vi "Dev List UI.vi"(8 "error in (no error)":errorcluster, 10 "stop event":refnum<user-event>, 11 "Operator UI in":refnum<class "Controller UI.lvclass">) -> (0 "error out":errorcluster)   [LabVIEW 2016, in "Controller UI.lvlib" / "Controller UI.lvclass"]
uses:
  <userlib>/Common Components/Controller UI/Controller UI.lvclass
  System.Windows.Forms
  C:/Program Files (x86)/National Instruments/LabVIEW 2016/vi.lib/ActorFramework/Actor/Actor.lvclass
  <userlib>/LabVIEWdotNetDataGrid/source/GridColumn/ColumnDefinition.ctl
  <userlib>/LabVIEWdotNetDataGrid/source/GridColumn/ColumnType.ctl
  <userlib>/Common Components/Controller UI/Controller UI.lvclass/Controller UI.ctl
  <vilib>/ActorFramework/Actor/Actor.lvclass/Actor.ctl
  <vilib>/ActorFramework/Message Enqueuer/Message Enqueuer.lvclass/Message Enqueuer.ctl
  <userlib>/Common Components/Hardware/DevInfo/DTColumn Index.ctl
  <userlib>/Common Components/Controller UI/Dev Variant Data.ctl
  <userlib>/Common Components/Hardware/DevInfo/DevInfo.lvclass
  <userlib>/Common Components/Controller UI/Update DT event data - checked out.ctl
  <userlib>/Common Components/Controller UI/Update DT event data - COMM status.ctl
  <userlib>/Common Components/Controller UI/DT Data File.ctl
  <userlib>/Common Components/Controller UI Messages/Write Selected DTRows Msg/Write Selected DTRows Msg.lvclass/Write Selected DTRows Msg.ctl
  <userlib>/Common Components/Controller Messages/Check Fcn and Dev Selection requested by UI Msg/Check Fcn and Dev Selection requested by UI Msg.lvclass/Check Fcn and Dev Selection requested by UI Msg.ctl
  <vilib>/Utility/error.llb/DialogType.ctl
  <userlib>/Common Components/Controller UI/Accessors/Read Update DT event.vi
  <userlib>/Common Components/Controller UI/Accessors/Read Function.vi
  <userlib>/Common Components/Controller UI/Accessors/Read Master_Slave.vi
  <vilib>/ActorFramework/Message Enqueuer/Init from Existing Queue.vi
  <vilib>/ActorFramework/Message Enqueuer/Enqueue.vi
  <userlib>/Common Components/Controller Messages/Check Fcn and Dev Selection requested by UI Msg/Check Fcn and Dev Selection requested by UI Msg.lvclass
  C:/Program Files (x86)/National Instruments/LabVIEW 2016/vi.lib/ActorFramework/Message/Message.lvclass
  <userlib>/Common Components/Controller UI Messages/Write Selected DTRows Msg/Write Selected DTRows Msg.lvclass
  <userlib>/Common Components/Controller Messages/Update Available COMM List Msg/Update Available COMM List Msg.lvclass
  <userlib>/LabVIEWdotNetDataGrid/source/DataGridView/Set DataCell (String).vi
  <vilib>/Utility/xml.llb/Read From XML File(string).vi
  <userlib>/LabVIEWdotNetDataGrid/source/DataGridView/Get DataArray (String).vi
  <vilib>/Utility/xml.llb/Write to XML File(string).vi
  <userlib>/LabVIEWdotNetDataGrid/source/DataGridView/Set ComboCell DataSource (String).vi
  <vilib>/ActorFramework/Message Priority Queue/Priority Enqueue.vi
  <vilib>/ActorFramework/Message Enqueuer/Message Enqueuer.lvclass
  <userlib>/LabVIEWdotNetDataGrid/source/DataGrid.lvlib
  <userlib>/LabVIEWdotNetDataGrid/source/Events/CellValueChanged/CellValueChanged.lvclass
  <userlib>/LabVIEWdotNetDataGrid/source/Events/CellClick/CellClick.lvclass
  <userlib>/LabVIEWdotNetDataGrid/source/Events/KeyDown/KeyDown.lvclass
  <userlib>/LabVIEWdotNetDataGrid/source/DataGridView/DataGridView.lvclass
  <userlib>/LabVIEWdotNetDataGrid/source/GridColumn/GridColumn.lvclass
  <vilib>/ActorFramework/Actor/Actor.lvclass
  <userlib>/LabVIEWdotNetDataGrid/source/DataTable/DataTable.lvclass
  <userlib>/Common Components/Common/Common.lvlib
  <userlib>/Common Components/Controller/Messages/Log Status/Log Status.lvclass
panel:
  in  "Refresh Button":bool
  in  "Down Button":bool
  in  "Up Button":bool
  in  "Remove Button":bool
  in  "Insert Button":bool
  in  "HW/DEV list":refnum<k24>(container)
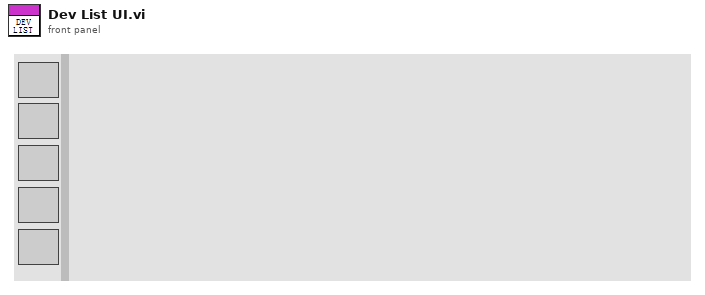
[diagram p1: front panel]
types:
  T1 = typedef "DataGrid.lvlib/GridColumn.lvclass/ColumnDefinition.ctl" = cluster{"name":string, "caption":string, "datatype":T2, "Params":string, "AutoSizeMode":i32, "FillWeight":sgl, "MinWidth":u32, "tooltip":string, "ReadOnly?":bool, "Visible?":bool}
  T2 = typedef "DataGrid.lvlib/GridColumn.lvclass/ColumnType.ctl" = enum16{"string", "image", "check", "numeric", "timestamp", "button", "combo", "link"}
  T3 = cluster{"registeredEvents":refnum<event-registration>, "Event Registration Refnum":refnum<event-registration>}
  T4 = typedef "Hardware.lvlib/DevInfo.lvclass/DTColumn Index.ctl" = enum16{"GUID", "Check", "Checked-out", "Status", "Device", "Label", "COMM", "Sub-COMM", "COMM Settings"}
  T5 = typedef "Controller UI.lvlib/Controller UI.lvclass/Update DT event data - checked out.ctl" = cluster{"GUID":string, "checked-out?":bool}
  T6 = typedef "Controller UI.lvlib/Controller UI.lvclass/Dev Variant Data.ctl" = cluster{"Row Index":i32, "DevInfo Obj":refnum<class "DevInfo.lvclass">}
  T7 = typedef "Controller UI.lvlib/Controller UI.lvclass/Update DT event data - COMM status.ctl" = cluster{"GUID":string, "COMM status":bool}
  T8 = typedef "Controller UI.lvlib/Controller UI.lvclass/DT Data File.ctl" = cluster{"ColumnSetup":T1[], "DataArray":string[][]}
  T9 = typedef "Controller UI.lvlib/Controller UI.lvclass/Update DT Cmd.ctl" = enum16{"Update HWtype\\HWplugin array", "Update Checked-out", "Update COMM Status", "Load DevInfo from File", "Save DevInfo to File", "Update COMM Address List"}
  T10 = typedef "DialogType.ctl" = u16
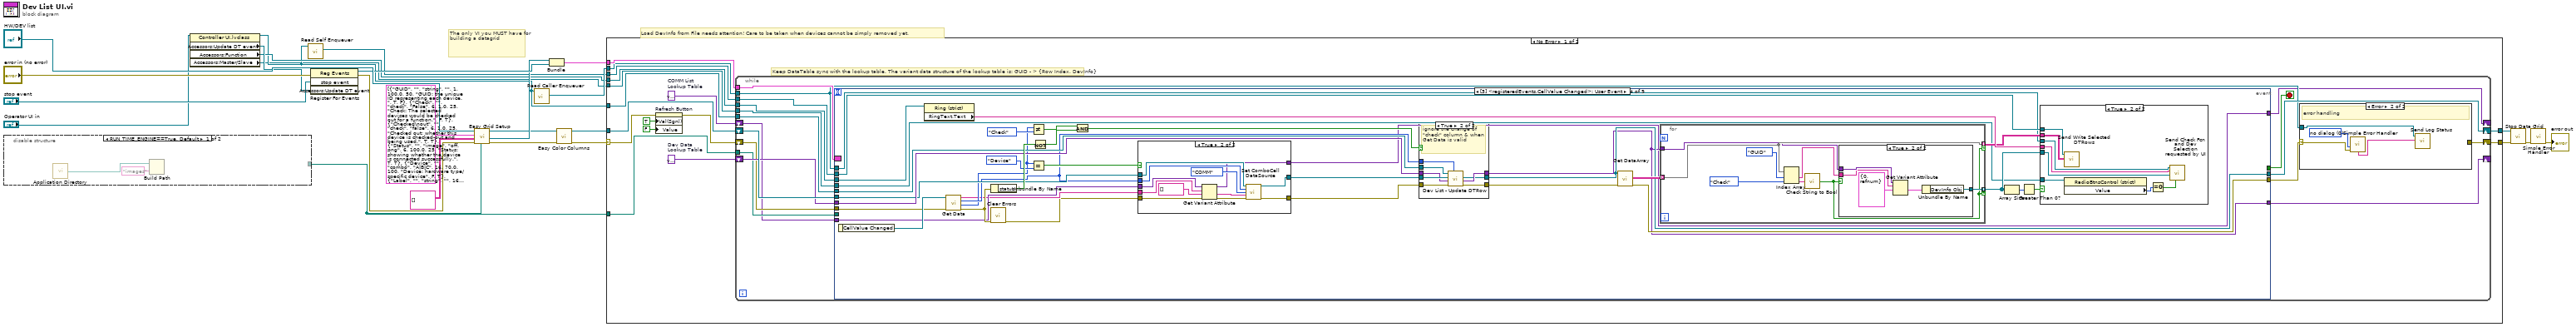
[diagram p0: block diagram]
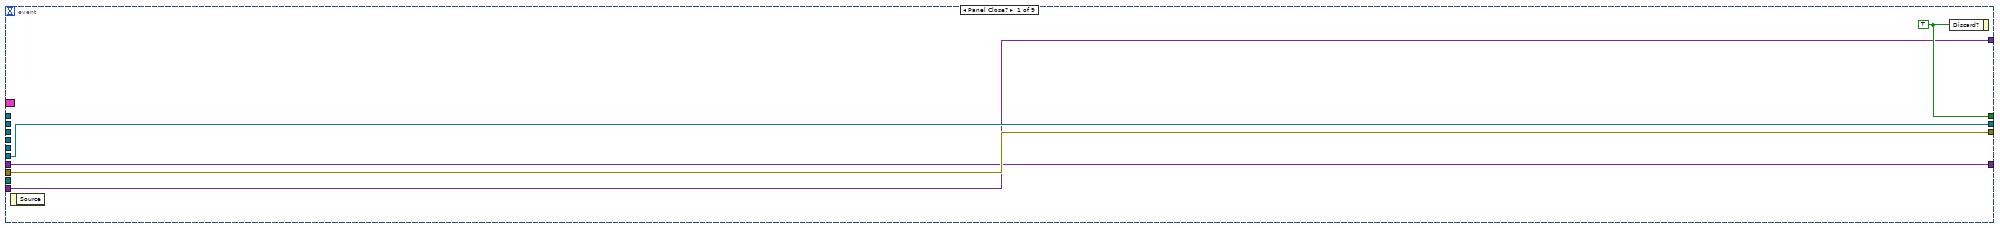
[diagram p3: hidden frame]
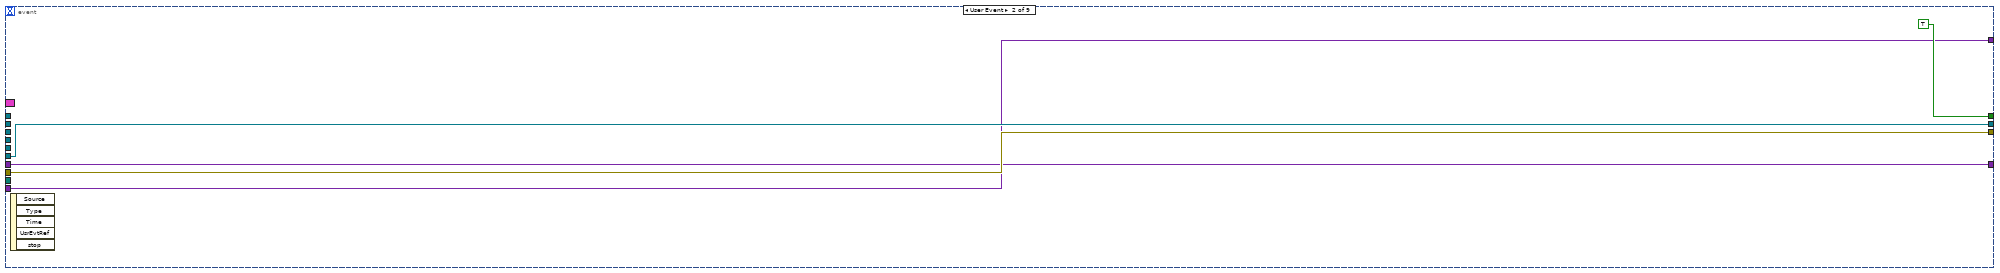
[diagram p4: hidden frame]
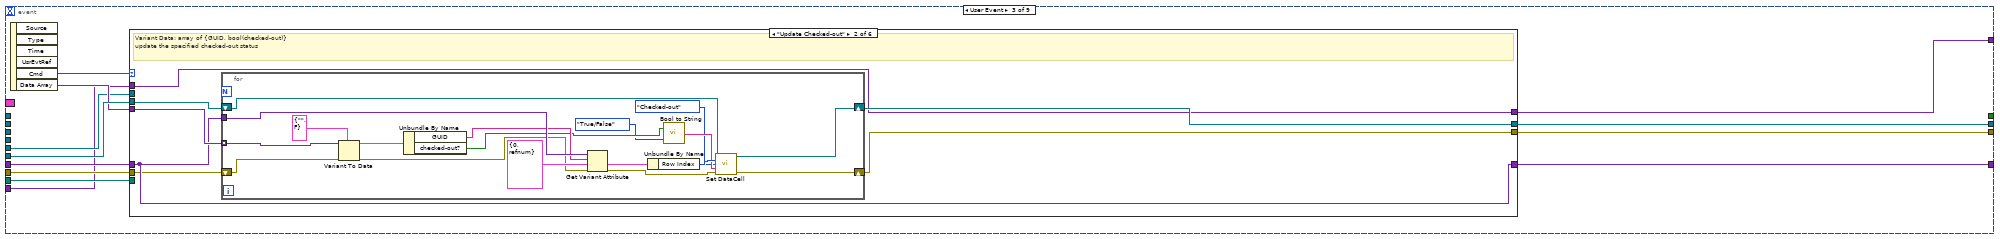
[diagram p5: hidden frame]
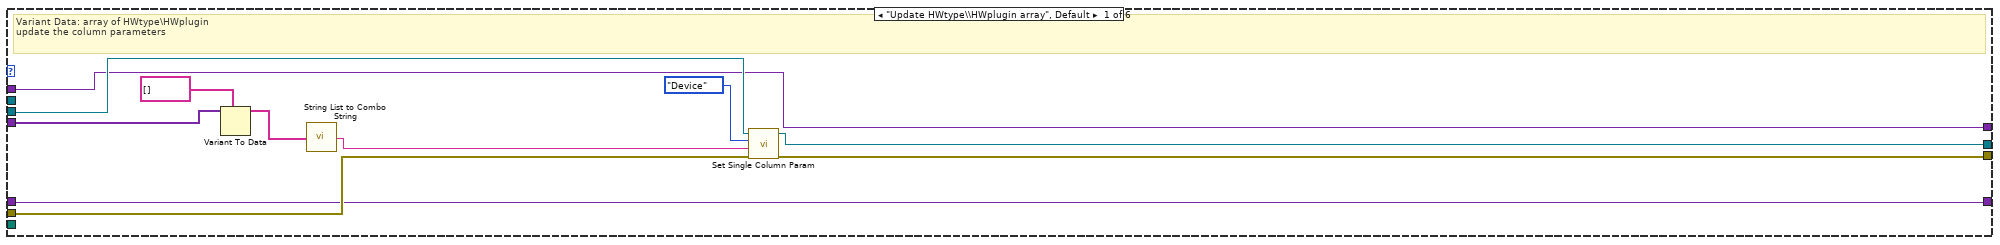
[diagram p6: hidden frame]
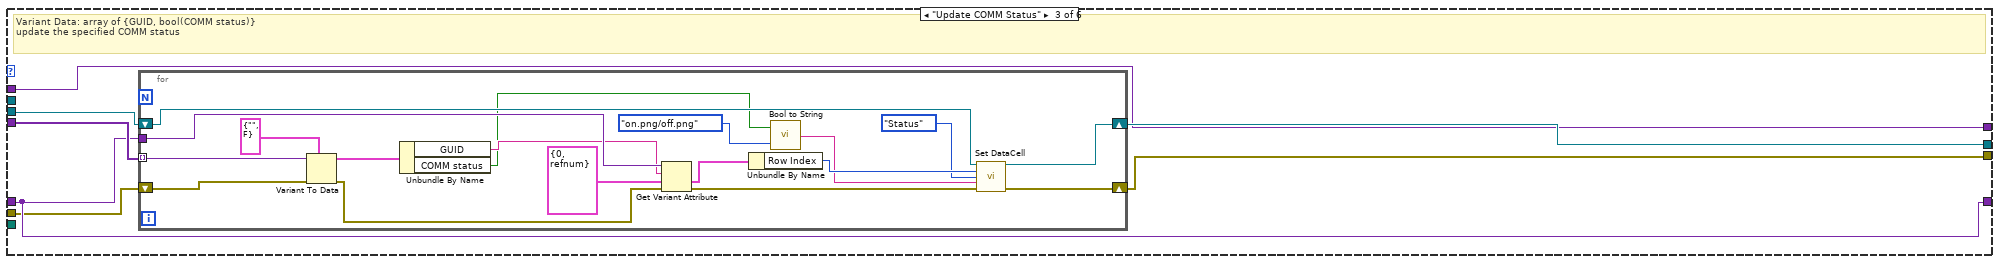
[diagram p7: hidden frame]
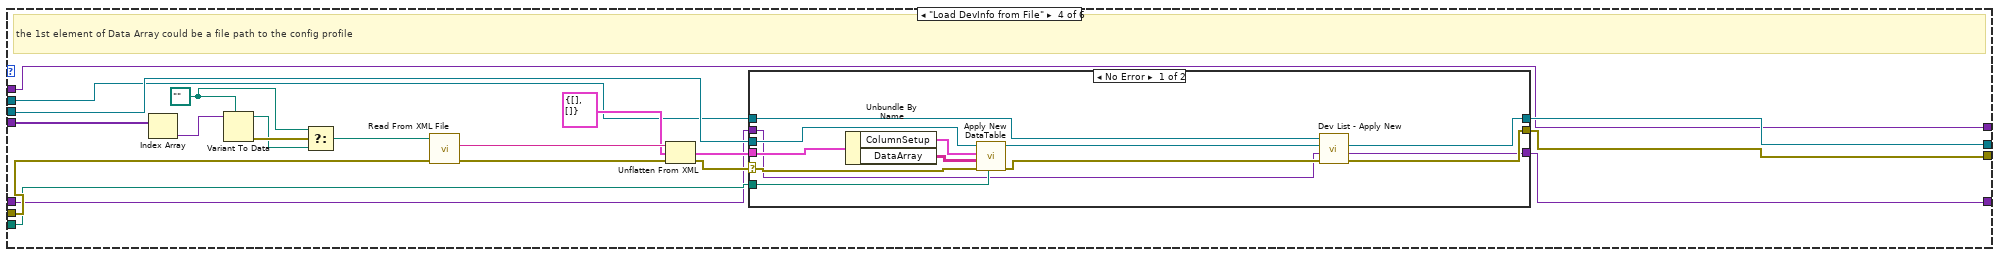
[diagram p8: hidden frame]
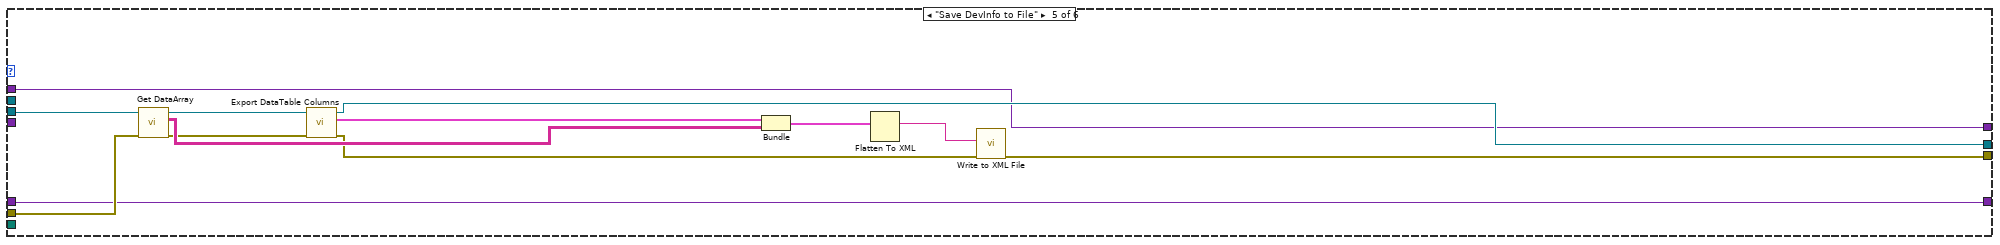
[diagram p10: hidden frame]
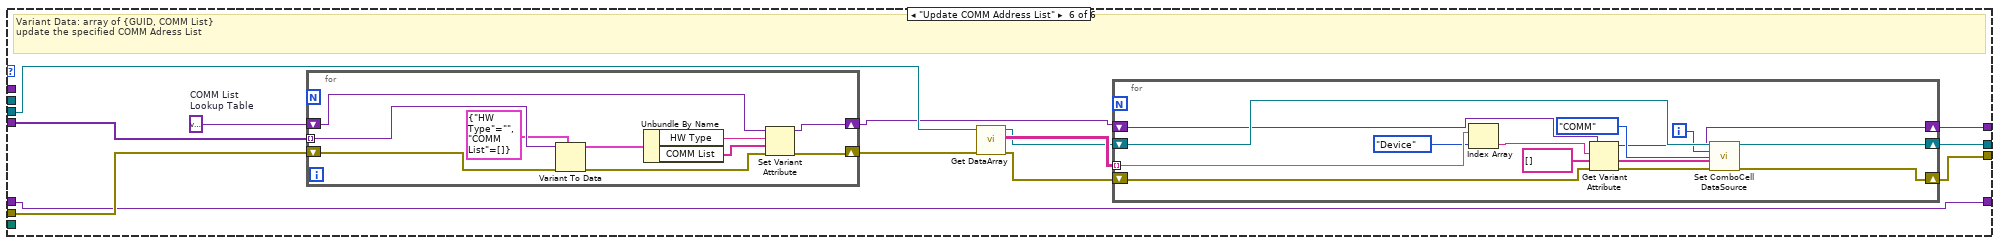
[diagram p11: hidden frame]
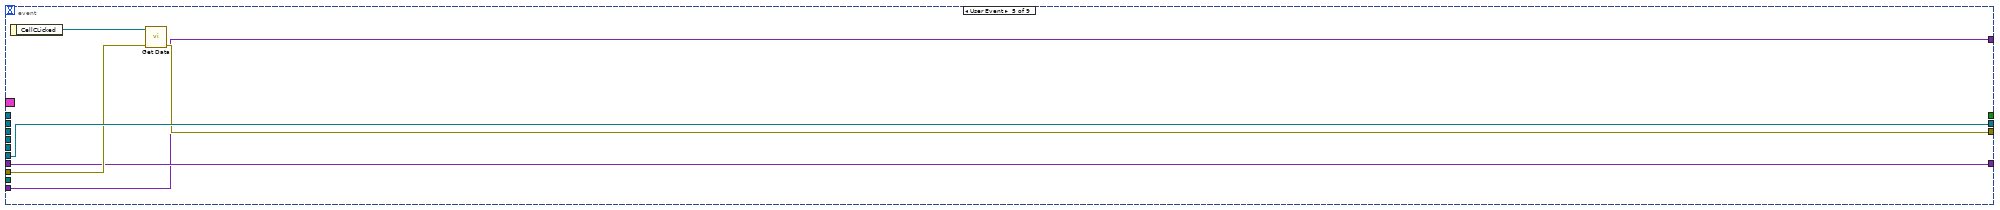
[diagram p16: hidden frame]
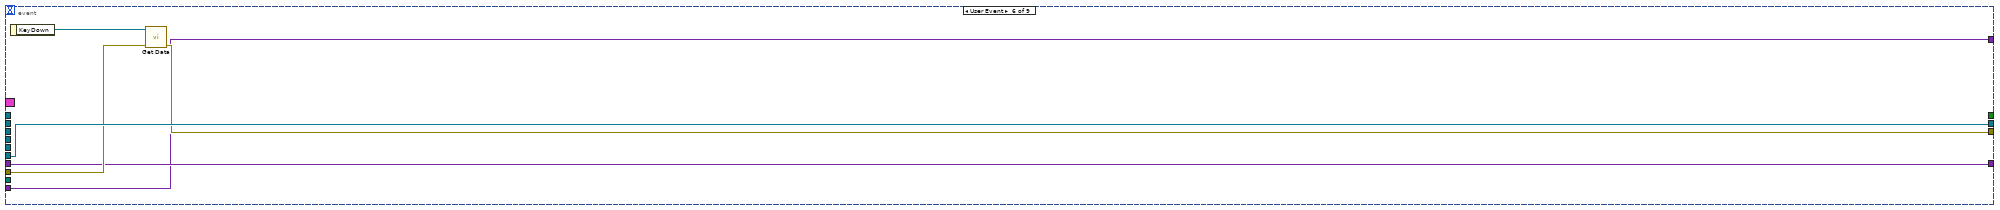
[diagram p17: hidden frame]
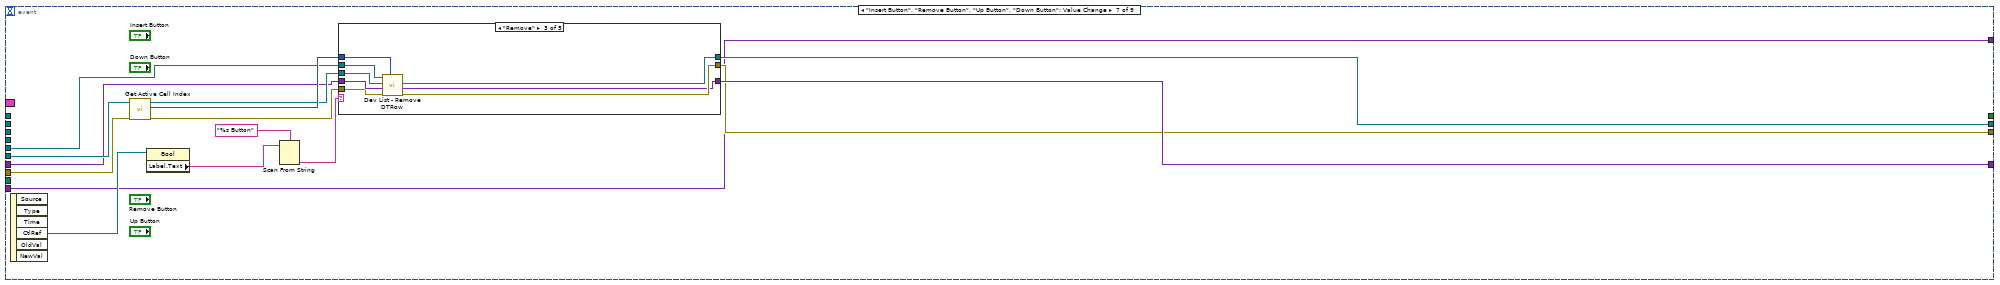
[diagram p18: hidden frame]
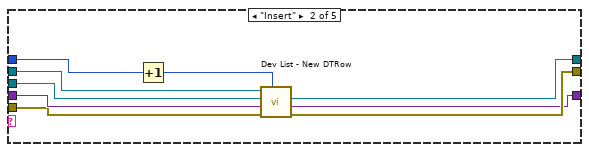
[diagram p20: hidden frame]
diagram:
  # "Load DevInfo from File needs attention! Care to be taken when devices cannot be simply removed yet."
  # "The only VI you MUST have for building a datagrid"
  n1 = disable-structure shown="RUN_TIME_ENGINE==True, Default" {
    disable-tunnel: [_ path "C:/Program Files (x86)/National Instruments/LabVIEW 2016/user.lib/LabVIEWdotNetDataGrid/images"] -> w2
    frame condition #0 {
      n2 = call <vilib>:"Application Directory.vi"() -> ("Application Directory"=w27:path)
      n3 = Build Path(base path=w27, name or relative path="images") -> ()  [unwired: 1 out]
    }
    frame condition #1 (active) {
    }
  }
  n4 = property class="Controller UI.lvclass"(reference="Operator UI in") -> (reference out=w6:refnum<class "Controller UI.lvclass">, "Accessors:Update DT event"=w9:refnum<user-event>, "Accessors:Function"=w7:refnum<vi>, "Accessors:Master/Slave"=w1:refnum<vi>)  [unwired: 1 in, 1 out]
  n5 = call <vilib>:"Read Self Enqueuer.vi"("Actor"=w6) -> ("Self Enqueuer"=w8:refnum<class "Message Enqueuer.lvclass">)  [unwired: 10 in]
  n6 = register-events(error in="error in (no error)", "stop event", w9) -> (reference out=w19:refnum<event-registration>, error out=w15:errorcluster)  [unwired: 1 in]
  n7 = call <userlib>:"Easy Grid Setup.vi"("Images Path"=w2, "error in"=w15, "DataSource Data"=string[][] [], "ColumnSetup"=T1[] [{"name"="GUID", "caption"="", "datatype"=enum."string", "Params"="", "AutoSizeMode"=1, "FillWeight"=100.0, "MinWidth"=50, "tooltip"="GUID: the unique ID representing each device.", "ReadOnly?"=TRUE, "Visible?"=FALSE}, {"name"="Check", "caption"="", "datatype"=enum."check", "Params"="False", "AutoSizeMode"=6, "FillWeight"=1.0, "MinWidth"=25, "tooltip"="Check: The selected devices would be checked out for a function.", "ReadOnly?"=FALSE, "Visible?"=TRUE}, {"name"="Checked\nout", "caption"="", "datatype"=enum."check", "Params"="false", "AutoSizeMode"=6, "FillWeight"=1.0, "MinWidth"=25, "tooltip"="Checked out: whether this device is checked-out and being used.", "ReadOnly?"=TRUE, "Visible?"=TRUE}, {"name"="Status", "caption"="", "datatype"=enum."image", "Params"="off.png", "AutoSizeMode"=6, "FillWeight"=100.0, "MinWidth"=25, "tooltip"="Status: showing whether the device is connected successfully.", "ReadOnly?"=TRUE, "Visible?"=TRUE}, {"name"="Device", "caption"="", "datatype"=enum."combo", "Params"="A|B|C", "AutoSizeMode"=16, "FillWeight"=70.0, "MinWidth"=100, "tooltip"="Device: hardware type/specific device", "ReadOnly?"=FALSE, "Visible?"=TRUE}, {"name"="Label", "caption"="", "datatype"=enum."string", "Params"="", "AutoSizeMode"=16, "FillWeight"=30.0, "MinWidth"=50, "tooltip"="Label: used as the alias in a running function, so multiple devices of the same abstract hardware type should have different labels in the same running function.", "ReadOnly?"=FALSE, "Visible?"=TRUE}, {"name"="COMM", "caption"="", "datatype"=enum."combo", "Params"="", "AutoSizeMode"=6, "FillWeight"=1.0, "MinWidth"=30, "tooltip"="COMM: the main communication port, e.g. COM, CAN ID, etc.", "ReadOnly?"=FALSE, "Visible?"=TRUE}, {"name"="Sub-\nCOMM", "caption"="", "datatype"=enum."numeric", "Params"="", "AutoSizeMode"=4, "FillWeight"=1.0, "MinWidth"=60, "tooltip"="Sub-COMM: address to the device if multiple connected to the main COMM.", "ReadOnly?"=FALSE, "Visible?"=TRUE}, {"name"="COMM\nSettings", "caption"="", "datatype"=enum."button", "Params"="", "AutoSizeMode"=6, "FillWeight"=1.0, "MinWidth"=20, "tooltip"="COMM Settings: clickable button if such settings available.", "ReadOnly?"=FALSE, "Visible?"=TRUE}], "DataGridView"="HW/DEV list") -> ("error out"=w25:errorcluster, "registeredEvents"=w18:refnum<event-registration>, "DataGrid out"=w5:refnum<class "DataGridView.lvclass">)  [unwired: 3 in, 1 out]
  n8 = call <vilib>:"Read Caller Enqueuer.vi"("Actor"=w6) -> ("Caller Enqueuer"=w11:refnum<class "Message Enqueuer.lvclass">)  [unwired: 10 in]
  n9 = Bundle("registeredEvents"=w18, "Event Registration Refnum"=w19) -> (w17:T3)  [unwired: 1 in]
  n10 = call <userlib>:"Easy Color Columns.vi"("error in (no error)"=w25, "DataGridView in"=w5) -> ("error out"=w4:errorcluster, "DataGridView out"=w24:refnum<class "DataGridView.lvclass">)  [unwired: 8 in]
  n11 = case shown="No Error" w4 {
    selector: w4 -> [w33 w382]
    tunnel: w24 -> [w44 w381]
    tunnel: [w43 w381] -> w23
    tunnel: w17 -> [w42 _]
    tunnel: [w41 w382] -> w3
    tunnel: w11 -> [w40 _]
    tunnel: w8 -> [w39 _]
    tunnel: w7 -> [w38 _]
    tunnel: w6 -> [w36 _]
    tunnel: w2 -> [w31 _]
    tunnel: w1 -> [w29 _]
    frame No Error {
      w30 = variant  # COMM List Lookup Table
      w37 = variant  # Dev Data Lookup Table
      # "Keep DataTable sync with the lookup table. The variant data structure of the lookup table is: GUID - > {Row Index, DevInfo}"
      n12 = property on="Refresh Button" class="Bool (strict)"(error in=w33, "Val(Sgnl)"=TRUE, "Value"=FALSE) -> (error out=w32:errorcluster)  [unwired: 1 in, 1 out]
      n13 = while {
        shift-right: [w60] -> w43
        shift-left: w44 -> [w61]
        tunnel: w42 -> [w59]
        tunnel: w40 -> [w48]
        tunnel: w39 -> [w57]
        tunnel: w38 -> [w56]
        shift-right: [w54] -> _
        shift-left: w37 -> [w55]
        tunnel: w36 -> [w53]
        shift-right: [w51] -> w41
        shift-left: w32 -> [w50]
        tunnel: w31 -> [w49]
        shift-right: [w46] -> _
        shift-left: w30 -> [w47]
        tunnel: w29 -> [w45]
        stop <- w58 stop-if-true
        n14 = event shown="[3] <registeredEvents.CellValue Changed>: User Event" {
          selector: w59 -> [_ _ _ _ _ _ _ _ _]
          dyn-events: _ -> [_ _ _ _ _ _ _ _ _]
          timeout: _ -> [_ _ _ _ _ _ _ _ _]
          tunnel: [w71 TRUE _ _ _ _ _ _ _] -> w58
          tunnel: w61 -> [w70 w76 w88 w246 w323 w329 w340 w375 w380]
          tunnel: [w70 w76 w85 w266 w323 w329 w338 w375 w380] -> w60
          tunnel: [w69 w75 w86 w263 w321 w327 w332 w373 w379] -> w52
          tunnel: w50 -> [w69 w75 w87 w269 w320 w326 w339 w373 w379]
          tunnel: w48 -> [_ _ _ w237 _ _ _ w371 _]
          tunnel: w57 -> [_ _ _ w268 _ _ _ _ _]
          tunnel: w56 -> [_ _ _ w265 _ _ _ _ _]
          tunnel: w55 -> [w68 w73 w82 w251 w319 w325 w335 w374 w378]
          tunnel: [w68 w73 w80 w249 w319 w325 w334 w374 w378] -> w54
          tunnel: w53 -> [_ _ w79 w250 _ _ w333 _ _]
          tunnel: w49 -> [_ _ w81 _ _ _ _ _ _]
          tunnel: w47 -> [w67 w72 w78 w243 w318 w324 w330 w372 w376]
          tunnel: [w67 w72 w77 w242 w318 w324 w330 w372 w376] -> w46
          tunnel: w45 -> [_ _ _ w236 _ _ _ _ _]
          event Panel Close? {
            w71 = TRUE ("Discard?")
            n15 = event-data() -> ()  [unwired: 1 in, 1 out]
            n16 = event-data("Discard?"=w71) -> ()  [unwired: 1 in, 1 out]
          }
          event User Event {
            n17 = event-data() -> ()  [unwired: 1 in, 5 out]
          }
          event User Event {
            n18 = event-data() -> ("Cmd"=w83:T9, "Data Array"=w84:variant[])  [unwired: 1 in, 4 out]
            n19 = case shown="\"Update Checked-out\"" w83 {
              tunnel: w88 -> [w99 w104 w129 w161 w198 w206]
              tunnel: w87 -> [w98 w102 w127 w166 w191 w211]
              tunnel: [w97 w101 w126 w163 w188 w199] -> w86
              tunnel: [w96 w103 w128 w162 w192 w203] -> w85
              tunnel: w84 -> [w95 w106 w131 w156 _ w210]
              tunnel: w82 -> [w90 w105 w130 w159 w187 w209]
              tunnel: w81 -> [_ _ _ w160 _ _]
              tunnel: [w90 w105 w130 w158 w187 w209] -> w80
              tunnel: w79 -> [_ _ _ w157 _ _]
              tunnel: w78 -> [w89 w100 w125 w150 w186 _]
              tunnel: [w89 w100 w125 w150 w186 w201] -> w77
              frame "Update HWtype\\HWplugin array", Default {
                # "Variant Data: array of HWtype\\HWplugin\nupdate the column parameters"
                n20 = Variant To Data(type=string[] [], Variant=w95) -> (data=w92:string[])  [unwired: 1 in, 1 out]
                n21 = call <userlib>:"String List to Combo String.vi"("find list"=w92) -> ("String"=w91:string)
                n22 = call <userlib>:"Set Single Column Param.vi"("error in (no error)"=w98, "Params"=w91, "column index"=DTColumn_Index."Device" ("DTColumn Index"), "DataGridView in"=w99) -> ("error out"=w97:errorcluster, "DataGridView out"=w96:refnum<class "DataGridView.lvclass">)  [unwired: 6 in]
              }
              frame "Update Checked-out" {
                # "Variant Data: array of {GUID, bool(checked-out)}\nupdate the specified checked-out status"
                n23 = for {
                  tunnel: w106 -> [w123] mode=indexing
                  tunnel: w105 -> [w124]
                  shift-right: [w118] -> w103
                  shift-left: w104 -> [w119]
                  shift-right: [w113] -> w101
                  shift-left: w102 -> [w111]
                  n24 = Variant To Data(error in=w111, type=T5 {"GUID"="", "checked-out?"=FALSE}, Variant=w123) -> (data=w112:T5, error out=w110:errorcluster)
                  n25 = Unbundle By Name(w112) -> ("GUID"=w122:string, "checked-out?"=w116:bool)
                  n26 = Get Variant Attribute(Variant=w124, name=w122, default value (empty Variant)=T6 {"Row Index"=0, "DevInfo Obj"=refnum} ("Dev Variant Data"), error in=w110) -> (value=w120:T6, error out=w114:errorcluster)  [unwired: 2 out]
                  n27 = Unbundle By Name(w120) -> ("Row Index"=w117:i32)
                  n28 = call <userlib>:"Bool to String.vi"("type (True/False)"=enum16{"True/False", "on.png/off.png"}."True/False", "Boolean"=w116) -> ("Bool String"=w115:string)
                  n29 = call-poly <userlib>:"Set DataCell.vi"("DataGridView in"=w119, "row index"=w117, "col index"=DTColumn_Index."Checked-out" ("DTColumn Index"), "Data"=w115, "error in"=w114) -> ("DataGridView out"=w118:refnum<class "DataGridView.lvclass">, "error out"=w113:errorcluster)  [unwired: 9 in]
                }
              }
              frame "Update COMM Status" {
                # "Variant Data: array of {GUID, bool(COMM status)}\nupdate the specified COMM status"
                n30 = for {
                  tunnel: w131 -> [w148] mode=indexing
                  tunnel: w130 -> [w149]
                  shift-right: [w143] -> w128
                  shift-left: w129 -> [w144]
                  shift-right: [w138] -> w126
                  shift-left: w127 -> [w136]
                  n31 = Variant To Data(error in=w136, type=T7 {"GUID"="", "COMM status"=FALSE} ("Cluster"), Variant=w148) -> (data=w137:T7, error out=w135:errorcluster)
                  n32 = Unbundle By Name(w137) -> ("GUID"=w147:string, "COMM status"=w141:bool)
                  n33 = Get Variant Attribute(Variant=w149, name=w147, default value (empty Variant)=T6 {"Row Index"=0, "DevInfo Obj"=refnum} ("Dev Variant Data"), error in=w135) -> (value=w145:T6, error out=w139:errorcluster)  [unwired: 2 out]
                  n34 = Unbundle By Name(w145) -> ("Row Index"=w142:i32)
                  n35 = call <userlib>:"Bool to String.vi"("type (True/False)"=enum16{"True/False", "on.png/off.png"}."on.png/off.png", "Boolean"=w141) -> ("Bool String"=w140:string)
                  n36 = call-poly <userlib>:"Set DataCell.vi"("DataGridView in"=w144, "row index"=w142, "col index"=DTColumn_Index."Status" ("DTColumn Index"), "Data"=w140, "error in"=w139) -> ("DataGridView out"=w143:refnum<class "DataGridView.lvclass">, "error out"=w138:errorcluster)  [unwired: 9 in]
                }
              }
              frame "Load DevInfo from File" {
                w152 = path "" ("XML File Path")
                # "the 1st element of Data Array could be a file path to the config profile"
                n37 = Index Array(array=w156) -> (element=w155:variant)  [unwired: 1 in]
                n38 = Variant To Data(type=w152, Variant=w155) -> (data=w153:path, error out=w154:errorcluster)  [unwired: 1 in]
                n39 = Select(t=w152, s=w154, f=w153) -> (s? t:f=w151:path)
                n40 = call-poly <vilib>:"Read From XML File.vi"("error in (no error)"=w166, "XML File Path"=w151) -> ("error out"=w165:errorcluster, "XML Elements"=w169:string)  [unwired: 7 in, 1 out]
                n41 = Unflatten From XML(xml string=w169, type=T8 {"ColumnSetup"=[], "DataArray"=[]} ("output cluster"), error in (no error)=w165) -> (value=w167:T8, error out=w164:errorcluster)
                n42 = case shown="No Error" w164 {
                  selector: w164 -> [w177 w184]
                  tunnel: w167 -> [w182 _]
                  tunnel: [w175 w184] -> w163
                  tunnel: [w173 w185] -> w162
                  tunnel: w161 -> [w179 w185]
                  tunnel: w160 -> [w178 _]
                  tunnel: w159 -> [w172 w183]
                  tunnel: [w171 w183] -> w158
                  tunnel: w157 -> [w170 _]
                  frame No Error {
                    n43 = Unbundle By Name(w182) -> ("ColumnSetup"=w181:T1[], "DataArray"=w180:string[][])
                    n44 = call <userlib>:"Apply New DataTable.vi"("Images Path"=w178, "error in (no error)"=w177, "DataArray"=w180, "ColumnSetup"=w181, "DataGridView in"=w179) -> ("error out"=w176:errorcluster, "DataGridView out"=w174:refnum<class "DataGridView.lvclass">)  [unwired: 5 in]
                    n45 = call <userlib>:"Dev List - Apply New.vi"("error in (no error)"=w176, "Dev Data Lookup Table in"=w172, "DataGridView in"=w174, "Controller UI in"=w170) -> ("error out"=w175:errorcluster, "Dev Data Lookup Table in out"=w171:variant, "DataGridView out"=w173:refnum<class "DataGridView.lvclass">)  [unwired: 5 in]
                  }
                  frame Error {
                  }
                }
              }
              frame "Save DevInfo to File" {
                n46 = call-poly <userlib>:"Get DataArray.vi"("error in (no error)"=w191, "DataGridView in"=w198) -> ("error out"=w190:errorcluster, "Array"=w195:string[][], "DataGridView out"=w197:refnum<class "DataGridView.lvclass">)  [unwired: 7 in]
                n47 = call <userlib>:"Export DataTable Columns.vi"("error in (no error)"=w190, "DataGridView in"=w197) -> ("error out"=w189:errorcluster, "ColumnSetup"=w196:T1[], "DataGridView out"=w192:refnum<class "DataGridView.lvclass">)  [unwired: 7 in]
                n48 = Bundle("ColumnSetup"=w196, "Array"=w195) -> (w194:cluster{"ColumnSetup":T1[], "Array":string[][]})  [unwired: 1 in]
                n49 = Flatten To XML(anything=w194) -> (xml string=w193:string)
                n50 = call-poly <vilib>:"Write to XML File.vi"("error in (no error)"=w189, "XML Input"=w193) -> ("error out"=w188:errorcluster)  [unwired: 7 in, 2 out]
              }
              frame "Update COMM Address List" {
                w207 = variant  # COMM List Lookup Table
                # "Variant Data: array of {GUID, COMM List}\nupdate the specified COMM Adress List"
                n51 = for {
                  tunnel: w210 -> [w234] mode=indexing
                  shift-right: [w232] -> w208
                  shift-left: w211 -> [w230]
                  shift-right: [w226] -> w202
                  shift-left: w207 -> [w235]
                  n52 = Variant To Data(error in=w230, type=cluster{"HW Type":string, "COMM List":string[]} {"HW Type"="", "COMM List"=[]} ("Cluster"), Variant=w234) -> (data=w231:cluster{"HW Type":string, "COMM List":string[]}, error out=w229:errorcluster)
                  n53 = Unbundle By Name(w231) -> ("HW Type"=w233:string, "COMM List"=w227:string[])
                  n54 = Set Variant Attribute(Variant=w235, name=w233, value=w227, error in=w229) -> (Variant out=w226:variant, error out=w232:errorcluster)  [unwired: 1 out]
                }
                n55 = call-poly <userlib>:"Get DataArray.vi"("error in (no error)"=w208, "DataGridView in"=w206) -> ("error out"=w200:errorcluster, "Array"=w205:string[][], "DataGridView out"=w204:refnum<class "DataGridView.lvclass">)  [unwired: 7 in]
                n56 = for {
                  tunnel: w205 -> [w221] mode=indexing
                  shift-right: [w224] -> w203
                  shift-left: w204 -> [w225]
                  shift-right: [w215] -> w201
                  shift-left: w202 -> [w219]
                  shift-right: [w212] -> w199
                  shift-left: w200 -> [w214]
                  i -> [w223]
                  n57 = Index Array(array=w221, index=DTColumn_Index."Device" ("DTColumn Index")) -> (element=w218:string)
                  n58 = Get Variant Attribute(Variant=w219, name=w218, default value (empty Variant)=string[] [] ("COMM List"), error in=w214) -> (duplicate Variant=w215:variant, value=w216:string[], error out=w213:errorcluster)  [unwired: 1 out]
                  n59 = call-poly <userlib>:"Set ComboCell DataSource.vi"("DataGridView in"=w225, "row index"=w223, "col index"=DTColumn_Index."COMM" ("DTColumn Index"), "Combo DataSource"=w216, "error in"=w213) -> ("DataGridView out"=w224:refnum<class "DataGridView.lvclass">, "error out"=w212:errorcluster)  [unwired: 9 in]
                }
              }
            }
          }
          event User Event {
            n60 = event-data() -> ("CellValue Changed"=w270:refnum<class "Abstract EVENT.lvclass">)  [unwired: 1 in]
            n61 = property class="Ring (strict)"(reference=w265) -> ("RingText.Text"=w264:string)  [unwired: 1 in, 2 out]
            n62 = call <userlib>:"Get Data.vi"("error in (no error)"=w269, "DataGrid.lvlib:Abstract EVENT.lvclass"=w270) -> ("error out"=w261:errorcluster, "column"=w244:i32, "row"=w245:i32, "cell value"=w241:string)  [unwired: 6 in]
            n63 = Unbundle By Name(w261) -> ("status"=w260:bool)
            n64 = call <vilib>:"Clear Errors.vi"("error in (no error)"=w261) -> ("error out"=w240:errorcluster)  [unwired: 5 in, 1 out]
            n65 = Not Equal?(x=w244, y=DTColumn_Index."Check" ("DTColumn Index")) -> (x != y?=w258:bool)
            n66 = Equal?(x=w244, y=DTColumn_Index."Device" ("DTColumn Index")) -> (x = y?=w247:bool)
            n67 = Not(x=w260) -> (.not. x?=w259:bool)
            n68 = And(x=w258, y=w259) -> (x .and. y?=w257:bool)
            n69 = case shown="True" w247 {
              tunnel: w246 -> [w271 w285]
              tunnel: w245 -> [_ w284]
              tunnel: w243 -> [w273 w282]
              tunnel: [w273 w281] -> w242
              tunnel: w241 -> [_ w280]
              tunnel: w240 -> [w272 w278]
              tunnel: [w271 w276] -> w239
              tunnel: [w272 w275] -> w238
              frame False {
              }
              frame True {
                n70 = Get Variant Attribute(Variant=w282, name=w280, default value (empty Variant)=string[] [] ("Combo DataSource"), error in=w278) -> (duplicate Variant=w281:variant, value=w274:string[], error out=w277:errorcluster)  [unwired: 1 out]
                n71 = call-poly <userlib>:"Set ComboCell DataSource.vi"("DataGridView in"=w285, "row index"=w284, "col index"=DTColumn_Index."COMM" ("DTColumn Index"), "Combo DataSource"=w274, "error in"=w277) -> ("DataGridView out"=w276:refnum<class "DataGridView.lvclass">, "error out"=w275:errorcluster)  [unwired: 9 in]
              }
            }
            n72 = case shown="True" w257 {
              tunnel: w239 -> [w309 w316]
              tunnel: w245 -> [_ w311]
              tunnel: w238 -> [w308 w313]
              tunnel: [w309 w310] -> w266
              tunnel: [w308 w312] -> w262
              tunnel: w251 -> [w307 w315]
              tunnel: [w307 w314] -> w249
              tunnel: w250 -> [_ w317]
              frame False {
              }
              frame True {
                # "ignore the change of \"check\" column & when Get Data is valid"
                n73 = call <userlib>:"Dev List - Update DTRow.vi"("Row Index"=w311, "error in (no error)"=w313, "Dev Data Lookup Table in"=w315, "DataGridView in"=w316, "Controller UI in"=w317) -> ("error out"=w312:errorcluster, "Dev Data Lookup Table in out"=w314:variant, "DataGridView out"=w310:refnum<class "DataGridView.lvclass">)  [unwired: 4 in]
              }
            }
            n74 = call-poly <userlib>:"Get DataArray.vi"("error in (no error)"=w262, "DataGridView in"=w266) -> ("error out"=w263:errorcluster, "Array"=w267:string[][])  [unwired: 7 in, 1 out]
            n75 = for {
              tunnel: w267 -> [w300] mode=indexing
              tunnel: [w300] -> w256 mode=indexing if=w298
              tunnel: [w299] -> w254 mode=indexing if=w298
              tunnel: w249 -> [w297]
              n76 = Index Array(array=w300, index #1=DTColumn_Index."GUID" ("DTColumn Index"), index #2=DTColumn_Index."Check" ("DTColumn Index")) -> (element #1=w296:string, element #2=w301:string)
              n77 = call <userlib>:"Check String to Bool.vi"("string of check"=w301) -> ("Boolean"=w298:bool)
              n78 = case shown="True" w298 {
                tunnel: [_ w303] -> w299
                tunnel: w297 -> [_ w306]
                tunnel: w296 -> [_ w305]
                frame False {
                }
                frame True {
                  n79 = Get Variant Attribute(Variant=w306, name=w305, default value (empty Variant)=T6 {"Row Index"=0, "DevInfo Obj"=refnum} ("Dev Variant Data")) -> (value=w302:T6)  [unwired: 1 in, 3 out]
                  n80 = Unbundle By Name(w302) -> ("DevInfo Obj"=w303:refnum<class "DevInfo.lvclass">)
                }
              }
            }
            n81 = Array Size(array=w254) -> (size(s)=w255:i32)
            n82 = Greater Than 0?(x=w255) -> (x > 0?=w253:bool)
            n83 = case shown="True" w253 {
              tunnel: w268 -> [_ w293]
              tunnel: w237 -> [_ w292]
              tunnel: w264 -> [_ w291]
              tunnel: w254 -> [_ w290]
              tunnel: w256 -> [_ w289]
              tunnel: w236 -> [_ w288]
              frame False {
              }
              frame True {
                n84 = call <userlib>:"Send Write Selected DTRows.vi"("Selected DTRows"=w289, "Message Enqueuer"=w293) -> ()  [unwired: 8 in, 2 out]
                n85 = property class="RadioBtnsControl (strict)"(reference=w288) -> ("Value"=w287:enum32{"Master", "Slave"})  [unwired: 1 in, 2 out]
                n86 = Equal To 0?(x=w287) -> (x = 0?=w286:bool)
                n87 = call <userlib>:"Send Check Fcn and Dev Selection requested by UI.vi"("Master?"=w286, "DevInfos"=w290, "Function Name"=w291, "Message Enqueuer"=w292) -> ()  [unwired: 6 in, 2 out]
              }
            }
          }
          event User Event {
            n88 = event-data() -> ("CellCLicked"=w322:refnum<class "Abstract EVENT.lvclass">)  [unwired: 1 in]
            n89 = call <userlib>:"Get Data.vi"("error in (no error)"=w320, "DataGrid.lvlib:Abstract EVENT.lvclass"=w322) -> ("error out"=w321:errorcluster)  [unwired: 7 in, 2 out]
          }
          event User Event {
            n90 = event-data() -> ("KeyDown"=w328:refnum<class "Abstract EVENT.lvclass">)  [unwired: 1 in]
            n91 = call <userlib>:"Get Data.vi"("error in (no error)"=w326, "DataGrid.lvlib:Abstract EVENT.lvclass"=w328) -> ("error out"=w327:errorcluster)  [unwired: 8 in, 1 out]
          }
          event "Insert Button", "Remove Button", "Up Button", "Down Button": Value Change {
            n92 = event-data() -> ("CtlRef"=w344:refnum<vi>)  [unwired: 1 in, 5 out]
            n93 = call <userlib>:"Get Active Cell Index.vi"("error in (no error)"=w339, "DataGridView in"=w340) -> ("error out"=w331:errorcluster, "RowIndex"=w337:i32, "DataGridView out"=w336:refnum<class "DataGridView.lvclass">)  [unwired: 6 in, 1 out]
            n94 = property class="Bool"(reference=w344) -> ("Label.Text"=w343:string)  [unwired: 1 in, 2 out]
            n95 = Scan From String(format string="%s Button", input string=w343) -> (output 1=w341:string)  [unwired: 3 in, 3 out]
            n96 = case shown="\"Remove\"" w341 {
              tunnel: w336 -> [w347 w355 w364 w367 w370]
              tunnel: [w347 w354 w359 w367 w370] -> w338
              tunnel: w337 -> [_ w356 w358 _ _]
              tunnel: [w346 w351 w361 w366 w369] -> w332
              tunnel: w331 -> [w346 w352 w362 w366 w369]
              tunnel: w335 -> [w345 w353 w363 w365 w368]
              tunnel: [w345 w350 w360 w365 w368] -> w334
              tunnel: w333 -> [_ w348 w357 _ _]
              frame Default {
              }
              frame "Insert" {
                n97 = Increment(x=w356) -> (x+1=w349:i32)
                n98 = call <userlib>:"Dev List - New DTRow.vi"("Row Index"=w349, "error in (no error)"=w352, "Dev Data Lookup Table in"=w353, "DataGridView in"=w355, "Controller UI in"=w348) -> ("error out"=w351:errorcluster, "Dev Data Lookup Table in out"=w350:variant, "DataGridView out"=w354:refnum<class "DataGridView.lvclass">)  [unwired: 4 in]
              }
              frame "Remove" {
                n99 = call <userlib>:"Dev List - Remove DTRow.vi"("Row Index"=w358, "error in (no error)"=w362, "Dev Data Lookup Table in"=w363, "DataGridView in"=w364, "Controller UI in"=w357) -> ("error out"=w361:errorcluster, "Dev Data Lookup Table in out"=w360:variant, "DataGridView out"=w359:refnum<class "DataGridView.lvclass">)  [unwired: 4 in]
              }
              frame "Up" {
              }
              frame "Down" {
              }
            }
          }
          event "Refresh Button": Value Change {
            n100 = event-data() -> ()  [unwired: 1 in, 6 out]
            n101 = call <userlib>:"Send Update Available COMM List.vi"("Message Enqueuer"=w371) -> ()  [unwired: 9 in, 2 out]
          }
          event "Refresh Button": Mouse Up {
            n102 = event-data() -> ()  [unwired: 1 in, 8 out]
            n103 = local write "Refresh Button"(FALSE) -> ()
          }
        }
        n104 = case shown="Error" w52 {
          selector: w52 -> [w62 w65]
          tunnel: w48 -> [_ w64]
          tunnel: [w62 _] -> w51
          frame No Error {
          }
          frame Error {
            w66 = T10 0 items=["no dialog", "OK message", "continue or stop message", "OK message + warnings", "continue/stop + warnings"] ("type of dialog (OK msg:1)")
            # "error handling"
            n105 = call <vilib>:"Simple Error Handler.vi"("type of dialog (OK msg:1)"=w66, "error in (no error)"=w65) -> ("message"=w63:string)  [unwired: 3 in, 4 out]
            n106 = call <userlib>:"Send Log Status.vi"("String"=w63, "Message Enqueuer in"=w64) -> ()  [unwired: 8 in, 2 out]
          }
        }
      }
    }
    frame Error {
    }
  }
  n107 = call <userlib>:"Stop Data Grid.vi"("error in (no error)"=w3, "DataGridView in"=w23) -> ("error out"=w22:errorcluster)  [unwired: 8 in, 1 out]
  n108 = call <vilib>:"Simple Error Handler.vi"("error in (no error)"=w22) -> ("error out"=→"error out":errorcluster)  [unwired: 4 in, 4 out]
